vi "stepNhold.vi"() -> ()   [LabVIEW 2025]
panel:
  in  "T control mode":u16(ring)=4 items=["Tprobe", "Tsorb", "Fast Tsweep", "Skip T stable", "open loop", "Janis CCR", "PPMS"]
  in  "Motor control":enum16{"BLM motor", "IMS motor"}(ring)
  in  "stop dataacq":bool
  in  "T0 336":refnum<visa-resource-name>="GPIB0::12::INSTR"
  out "waiting (s)":dbl
  in  "meas time (s)":dbl=10.0
  in  "rate(T/min)":dbl=0.3 min=0.0
  in  "Power supply":T1(ring)
  in  "Exp. Mode":u16(ring)=1 items=["T sweep", "H sweep", "Angle sweep", "Other"]
  in  "Pass":bool
  in  "NML Data Acquisition VI":string(combo)="NML Data Acquisition-New.vi"
  out "stable":bool
  out "Reading":dbl=-999.99 format="%#_4g"
  out "done":i32
  in  "Finish":bool
  out "On Target":bool=TRUE
  in  "Target error":dbl=0.002 format="%#_13g"
  in  "timeout (s)":dbl=600.0
  out "time passed (s)":dbl format="%#_4g"
  out "status":string="Temp reached. Wait for stability"
  out "completed":bool
  out "table":dbl[][](array[numeric])=[[0.01, 0.41], [0.05, 0.32], [0.1, 0.33], [6.0, 2.0], [8.0, 2.0], [10.0, 2.0], [14.0, 2.0], [15.0, 2.0], [16.0, 2.0], [17.0, 2.0], [18.0, 2.0], [19.0, 2.0], [20.0, 2.0], [21.0, 2.0], [25.0, 1.0], [26.0, 2.0], [28.0, 2.0], [30.0, 2.0], [28.0, 2.0], [26.0, 2.0], [25.0, 2.0], [21.0, 1.0], [20.0, 2.0], [19.0, 2.0], [18.0, 2.0], [17.0, 2.0], [16.0, 2.0], [15.0, 2.0], [14.0, 2.0], [11.0, 1.0], [10.0, 2.0], [8.0, 2.0], [6.0, 2.0], [4.0, 2.0], [2.0, 2.0], [0.0, 2.0]]
  in  "Set T, wait (m)":string="0.01 0.41\n0.05 0.32\n0.1 0.33\n6 2\n8 2\n10 2\n14 2\n15 2\n16 2\n17 2\n18 2\n19 2\n20 2\n21 2\n25 1\n26 2\n28 2\n30 2\n28 2\n26 2\n25 2\n21 1\n20 2\n19 2\n18 2\n17 2\n16 2\n15 2\n14 2\n11 1\n10 2\n8 2\n6 2\n4 2\n2 2\n0 2" caption="Set Field(T), rate(T/min) (defualt rate: first row value)"
  in  "Use\nTable":bool
  in  "stable wait":dbl=10.0
  out "Target value":dbl=-1000.0
  in  "step":dbl=0.05
  in  "Final Target":dbl=1.0
  in  "Initial Target":dbl
  # "Step and Hold temperature, field or angle.\nData will be collected only when 'hold' state.\n\nField and Angle: There is no stability check\nTemp: Tcheck.vi check the stability.\n\nTiming\nstable wait: waiting time after 'hold' condition is met.\nmeas time (s): duration for data collection.\ntimeout (s): max time allowed to reach 'hold' condition."
  # "(s)"
  # "If ON, when the final target is reached,\ndata acq will be stopped\nand the data will be saved\n\nOtherwise, it will be paused."
  # "Txb: T's (0, hot, col) with heater off\nTxh: T's with heater on"
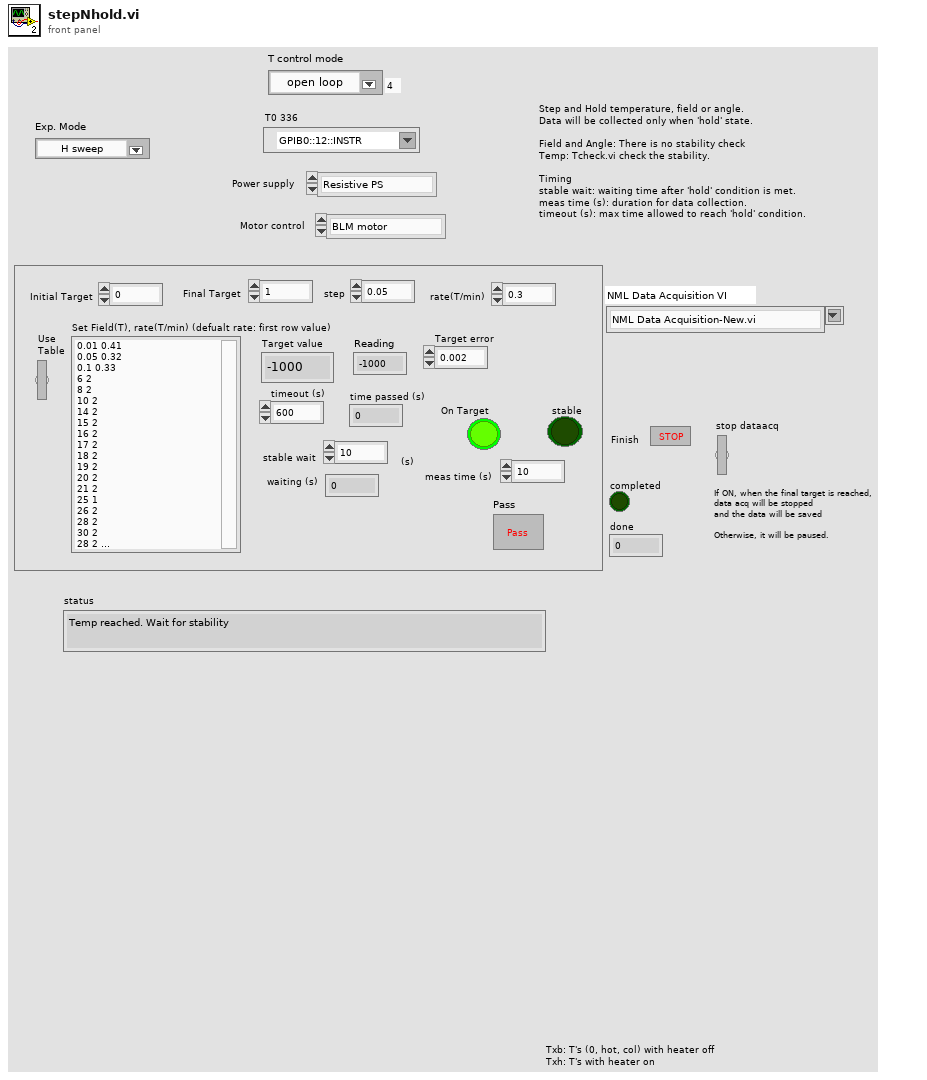
[diagram p1: front panel]
types:
  T1 = enum16{"Resistive PS", "SCM2 PS", "SCM1 PS", "Generic PS", "PPMS"}
  T2 = enum32{"New", "Stop", "Trigger", "Delta Trigger", "Run", "Pause"}
  T3 = enum32{"New", "Stop", "Trigger", "Delta Trigger", "Run", "Pause", "comments", "Started?"}
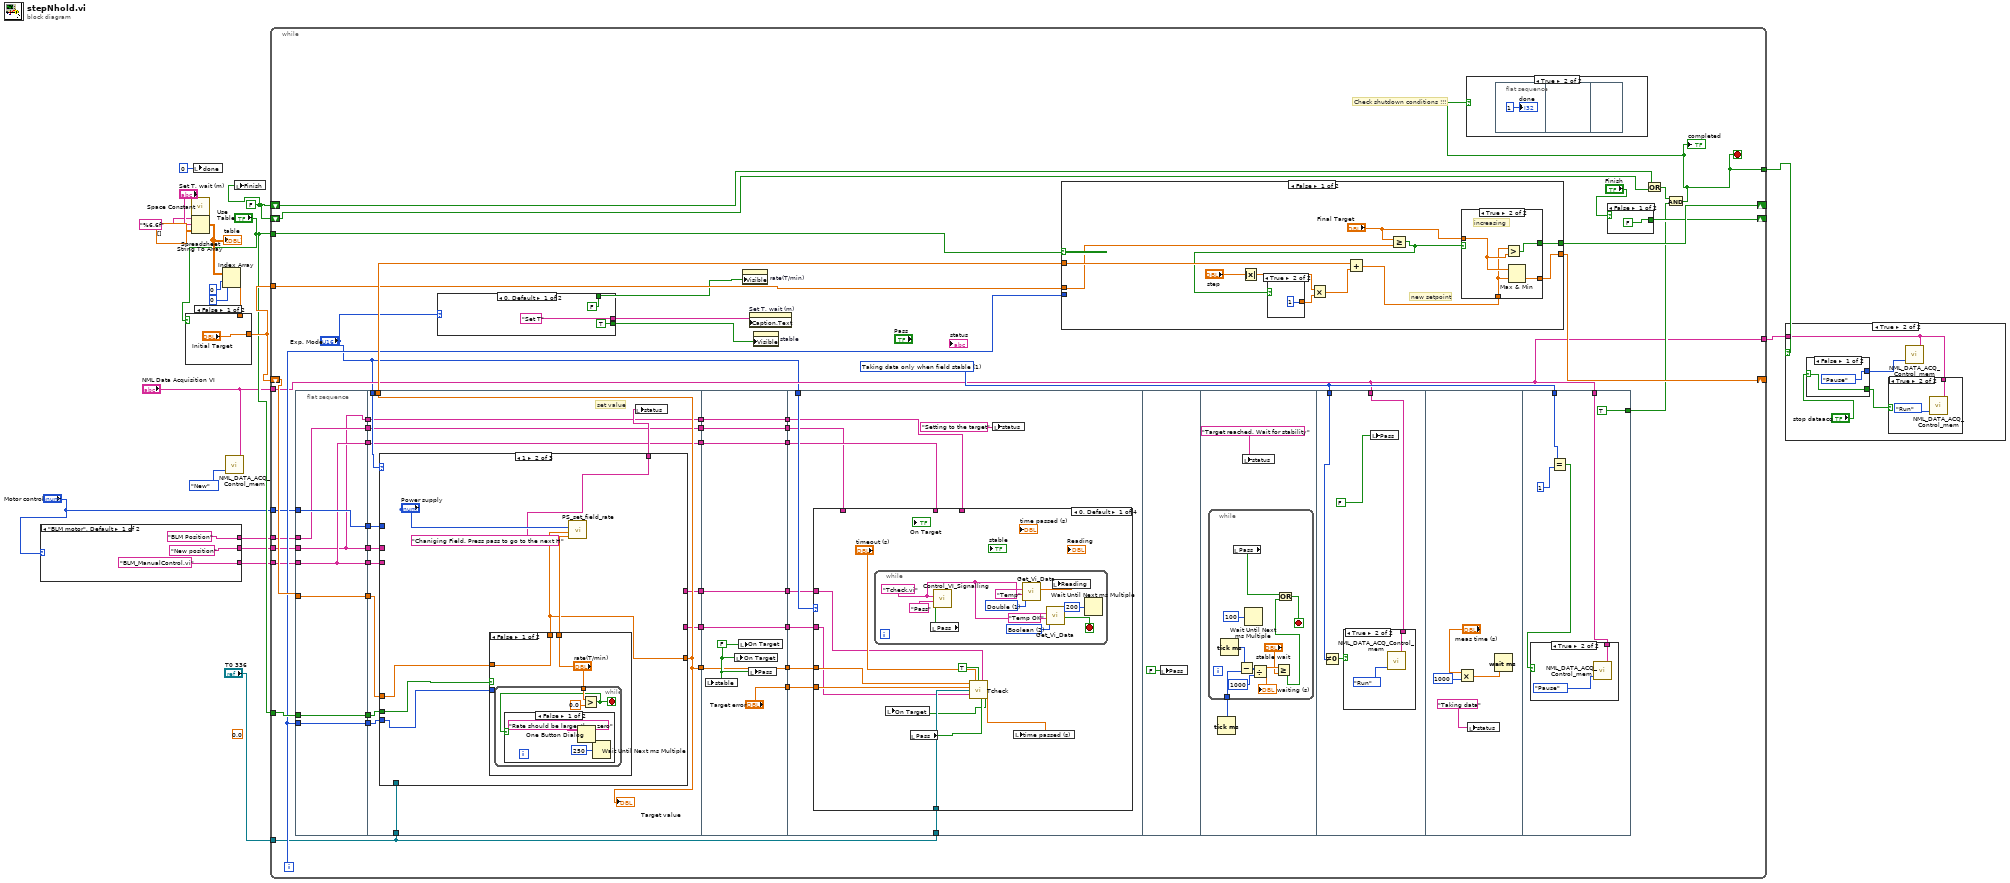
[diagram p0: block diagram]
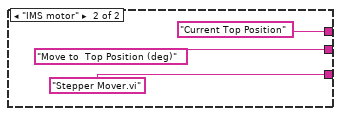
[diagram p2: hidden frame]
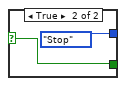
[diagram p5: hidden frame]
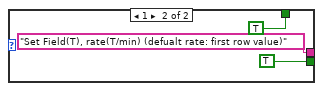
[diagram p7: hidden frame]
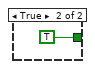
[diagram p9: hidden frame]
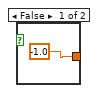
[diagram p10: hidden frame]
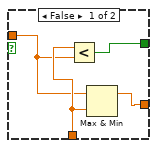
[diagram p11: hidden frame]
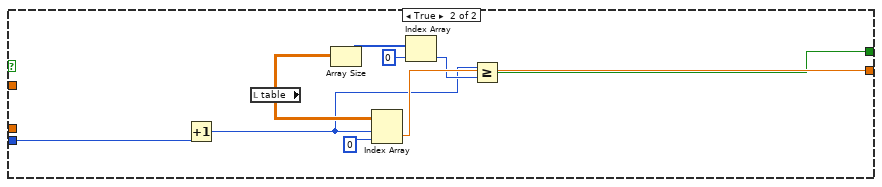
[diagram p12: hidden frame]
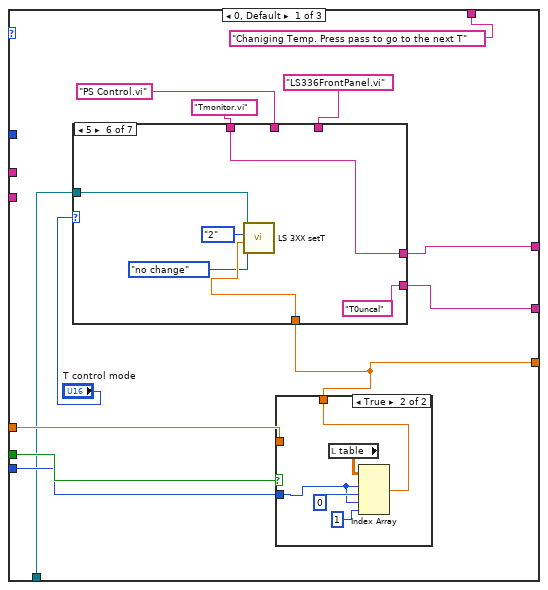
[diagram p13: hidden frame]
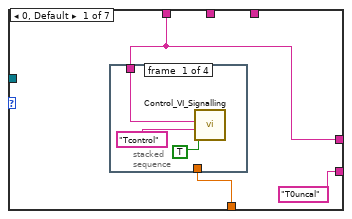
[diagram p14: hidden frame]
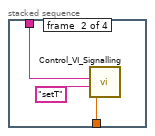
[diagram p15: hidden frame]
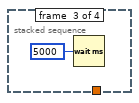
[diagram p16: hidden frame]
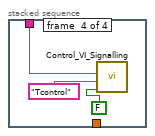
[diagram p17: hidden frame]
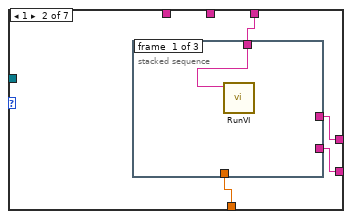
[diagram p18: hidden frame]
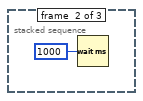
[diagram p19: hidden frame]
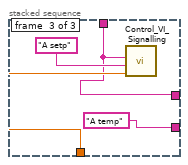
[diagram p20: hidden frame]
diagram:
  (unwired) 0.0 ("setT")
  w11 = FALSE
  n1 = case shown="\"BLM motor\", Default" "Motor control" {
    tunnel: ["BLM_ManualControl.vi" ("Target VI name") "Stepper Mover.vi" ("Target VI name")] -> w5
    tunnel: ["New position" ("Control Name") "Move to  Top Position (deg)" ("Control Name")] -> w4
    tunnel: ["BLM Position" "Current Top Position"] -> w2
    frame "BLM motor", Default {
    }
    frame "IMS motor" {
    }
  }
  n2 = call <vilib>:"Space Constant.vi"() -> ("String"=w17:string)
  n3 = Spreadsheet String To Array(delimiter (Tab)=w17, format string="%6.6f", spreadsheet string="Set T, wait (m)", array type (2D Dbl)=dbl[][] []) -> (array=w16:dbl[][])
  "table" <- w16
  n4 = local write "done"(0 ("done")) -> ()
  n5 = Index Array(array=w16, index (row)=0, index (col)=0 ("disabled index (col)")) -> (element=w13:dbl)
  n6 = case shown="False" "Use\nTable" {
    tunnel: ["Initial Target" w29] -> w21
    tunnel: w13 -> [_ w29]
    frame False {
    }
    frame True {
    }
  }
  n7 = call "NML_DATA_ACQ_Control_mem.vi"("Enum"=T2."New", "NML Data Acquisition VI"="NML Data Acquisition VI") -> ()  [unwired: 4 in, 1 out]
  n8 = local write "Finish"(w11) -> ()
  n9 = while {
    shift-right: [w75] -> _
    shift-left: w21 -> [w77]
    tunnel: w21 -> [w74]
    tunnel: "Use\nTable" -> [w73]
    tunnel: "Use\nTable" -> [w72]
    shift-right: [w70] -> _
    shift-left: w11 -> [w66]
    shift-right: [w67] -> _
    shift-left: w11 -> [w65]
    tunnel: "NML Data Acquisition VI" -> [w54]
    tunnel: [w55] -> w7
    tunnel: [w54] -> w6
    tunnel: w5 -> [w50]
    tunnel: w4 -> [w49]
    tunnel: "Motor control" -> [w46]
    tunnel: w2 -> [w42]
    tunnel: "T0 336" -> [w34]
    i -> [w71]
    stop <- w55 stop-if-true
    w69 = u16 1 items=["No interrupt", "Taking data only when field stable", "Taking data always"] ("Data acqusition ? (Run and Pause)")
    # "Check shutdown conditions !!!"
    n10 = flat-sequence {
      tunnel: w71 -> [w121]
      tunnel: w72 -> [w122]
      tunnel: w77 -> [w123]
      tunnel: [w123] -> w58
      tunnel: [w122] -> w57
      tunnel: [w121] -> w56
      tunnel: [w119] -> w51
      tunnel: w50 -> [w119]
      tunnel: w49 -> [w117]
      tunnel: [w117] -> w48
      tunnel: [w120] -> w47
      tunnel: w46 -> [w120]
      tunnel: [w119] -> w43
      tunnel: w42 -> [w118]
      tunnel: [w118] -> w41
      tunnel: [w117] -> w36
      tunnel: [w132] -> w76
      tunnel: "Exp. Mode" -> [w134]
      tunnel: w58 -> [w136]
      tunnel: w57 -> [w138]
      tunnel: w56 -> [w137]
      tunnel: w34 -> [w133]
      tunnel: [w132] -> w53
      tunnel: w51 -> [w131]
      tunnel: w48 -> [w130]
      tunnel: w47 -> [w129]
      tunnel: [w128] -> w44
      tunnel: w43 -> [w128]
      tunnel: w41 -> [w127]
      tunnel: [w127] -> w40
      tunnel: [w126] -> w37
      tunnel: w36 -> [w126]
      tunnel: [w125] -> w33
      tunnel: [w124] -> w31
      tunnel: ["Target error"] -> w64
      tunnel: w53 -> [w270]
      tunnel: [w270] -> w52
      tunnel: [w269] -> w45
      tunnel: w44 -> [w269]
      tunnel: w40 -> [w268]
      tunnel: [w268] -> w39
      tunnel: [w267] -> w38
      tunnel: w37 -> [w267]
      tunnel: w33 -> [w266]
      tunnel: [w266] -> w32
      tunnel: w31 -> [w265]
      tunnel: [w265] -> w30
      tunnel: "Exp. Mode" -> [w282]
      tunnel: w64 -> [w281]
      tunnel: w52 -> [w279]
      tunnel: w45 -> [w278]
      tunnel: w39 -> [w277]
      tunnel: w38 -> [w276]
      tunnel: w34 -> [w275]
      tunnel: w32 -> [w274]
      tunnel: w30 -> [w273]
      tunnel: w69 -> [w362]
      tunnel: w54 -> [w361]
      tunnel: w69 -> [w375]
      tunnel: [TRUE] -> w59
      tunnel: w54 -> [w371]
      frame #0 {
      }
      frame #1 {
        # "set value"
        n11 = case shown="1" w134 {
          tunnel: w138 -> [w150 w215 w246]
          tunnel: w137 -> [w149 w218 w247]
          tunnel: w136 -> [w148 w214 w245]
          tunnel: [w144 w213 w243] -> w132
          tunnel: ["Chaniging Temp. Press pass to go to the next T" ("status") "Chaniging Field. Press pass to go to the next H" ("status") "Chaniging angle. Press pass to go to the next angle" ("status")] -> w135
          tunnel: w133 -> [w143 _ _]
          tunnel: w131 -> [_ _ w241]
          tunnel: w130 -> [_ _ w240]
          tunnel: w129 -> [_ _ w239]
          tunnel: [w140 _ _] -> w125
          tunnel: [w139 _ _] -> w124
          frame 0, Default {
            n12 = case shown="True" w150 {
              tunnel: [w206 w210] -> w144
              tunnel: w149 -> [_ w208]
              tunnel: w148 -> [w206 _]
              frame False {
              }
              frame True {
                n13 = local read "table"() -> (w211:dbl[][])
                n14 = Index Array(array=w211, index (row) #1=w208, index (col) #1=0 ("disabled index (row)"), index (row) #2=w208, index (col) #2=1 ("disabled index (col)")) -> (element #1=w210:dbl)  [unwired: 1 out]
              }
            }
            n15 = case shown="5" "T control mode" {
              tunnel: w144 -> [w151 w167 _ _ w175 w193 w199]
              tunnel: ["T0uncal" ("VI name") w166 _ _ "T0uncal" ("VI name") "T0uncal" ("VI name") w198] -> w139
              tunnel: "Tmonitor.vi" ("VI name") -> [w152 _ _ _ w174 w194 _]
              tunnel: [w152 w165 _ _ w174 w194 w197] -> w140
              tunnel: "LS336FrontPanel.vi" ("Target VI name") -> [_ w164 _ _ _ _ _]
              tunnel: w143 -> [_ _ _ _ _ w191 _]
              tunnel: "PS Control.vi" ("VI name") -> [_ _ _ _ _ _ w196]
              frame 0, Default {
                n16 = stacked-sequence {
                  tunnel: w152 -> [w155 w158 _ w163]
                  tunnel: w151 -> [_ w157 _ _]
                  frame #0 {
                    n17 = call "Control_VI_Signalling.vi"("Input Value"=TRUE ("Pass"), "Control Name"="Tcontrol", "Target VI name"=w155) -> ()  [unwired: 8 in, 1 out]
                  }
                  frame #1 {
                    n18 = call "Control_VI_Signalling.vi"("Input Value"=w157, "Control Name"="setT", "Target VI name"=w158) -> ()  [unwired: 8 in, 1 out]
                  }
                  frame #2 {
                    n19 = Wait (ms)(milliseconds to wait=u32 5000) -> ()  [unwired: 1 out]
                  }
                  frame #3 {
                    n20 = call "Control_VI_Signalling.vi"("Input Value"=FALSE ("Pass"), "Control Name"="Tcontrol", "Target VI name"=w163) -> ()  [unwired: 8 in, 1 out]
                  }
                }
              }
              frame 1 {
                n21 = stacked-sequence {
                  tunnel: w167 -> [_ _ w172]
                  tunnel: [_ _ "A temp" ("VI name")] -> w166
                  tunnel: [_ _ w170] -> w165
                  tunnel: w164 -> [w168 _ w170]
                  frame #0 {
                    n22 = call "RunVI.vi"("String"=w168) -> ()  [unwired: 10 in, 1 out]
                  }
                  frame #1 {
                    n23 = Wait (ms)(milliseconds to wait=u32 1000) -> ()  [unwired: 1 out]
                  }
                  frame #2 {
                    n24 = call "Control_VI_Signalling.vi"("Input Value"=w172, "Control Name"="A setp", "Target VI name"=w170) -> ()  [unwired: 8 in, 1 out]
                  }
                }
              }
              frame 2 {
              }
              frame 3 {
              }
              frame 4 {
                n25 = stacked-sequence {
                  tunnel: w174 -> [w177 w181 w184 _ w188]
                  tunnel: w175 -> [w178 _ _ _ _]
                  frame #0 {
                    n26 = call "Control_VI_Signalling.vi"("Input Value"=w178, "Control Name"="mc current", "Target VI name"=w177) -> ()  [unwired: 8 in, 1 out]
                  }
                  frame #1 {
                    n27 = call "Control_VI_Signalling.vi"("Input Value"=1 ("disabled index (col)"), "Control Name"="control mode", "Target VI name"=w181) -> ()  [unwired: 8 in, 1 out]
                  }
                  frame #2 {
                    n28 = call "Control_VI_Signalling.vi"("Input Value"=TRUE ("Pass"), "Control Name"="Tcontrol", "Target VI name"=w184) -> ()  [unwired: 8 in, 1 out]
                  }
                  frame #3 {
                    n29 = Wait (ms)(milliseconds to wait=u32 4000) -> ()  [unwired: 1 out]
                  }
                  frame #4 {
                    n30 = call "Control_VI_Signalling.vi"("Input Value"=FALSE ("Pass"), "Control Name"="Tcontrol", "Target VI name"=w188) -> ()  [unwired: 8 in, 1 out]
                  }
                }
              }
              frame 5 {
                n31 = call "LS 3XX setT.vi"("power"=enum16{"no change", "off", "low", "med", "high"}."no change", "setT"=w193, "loop"=enum16{"1", "2"}."2", "GPIB"=w191) -> ()  [unwired: 8 in]
              }
              frame 6 {
                n32 = stacked-sequence {
                  tunnel: w199 -> [_ _ w204]
                  tunnel: [_ _ "Tppms" ("VI name")] -> w198
                  tunnel: [_ _ w202] -> w197
                  tunnel: w196 -> [w200 _ w202]
                  frame #0 {
                    n33 = call "RunVI.vi"("String"=w200) -> ()  [unwired: 10 in, 1 out]
                  }
                  frame #1 {
                    n34 = Wait (ms)(milliseconds to wait=u32 1000) -> ()  [unwired: 1 out]
                  }
                  frame #2 {
                    n35 = call "Control_VI_Signalling.vi"("Input Value"=w204, "Control Name"="set T", "Target VI name"=w202) -> ()  [unwired: 8 in, 1 out]
                  }
                }
              }
            }
          }
          frame 1 {
            n36 = case shown="False" w215 {
              tunnel: ["rate(T/min)" w227] -> w216
              tunnel: w218 -> [_ w232]
              tunnel: [w220 w230] -> w213
              tunnel: w214 -> [w220 _]
              frame False {
                n37 = while {
                  tunnel: "rate(T/min)" -> [w223]
                  stop <- w221 stop-if-true
                  n38 = Greater?(x=w223, y=0.0) -> (0:w221:bool)
                  n39 = case shown="False" w221 {
                    frame False {
                      n40 = One Button Dialog(message="Rate should be larger than zero") -> ()  [unwired: 1 in, 1 out]
                      n41 = Wait Until Next ms Multiple(millisecond multiple=u32 250) -> ()  [unwired: 1 out]
                    }
                    frame True {
                    }
                  }
                }
              }
              frame True {
                n42 = local read "table"() -> (w226:dbl[][])
                n43 = Index Array(array=w226, index (row) #1=w232, index (col) #1=0 ("disabled index (row)"), index (row) #2=w232, index (col) #2=1 ("disabled index (col)")) -> (element #1=w230:dbl, element #2=w228:dbl)
                n44 = Not Equal To 0?(x=w228) -> (x != 0?=w229:bool)
                n45 = case shown="False" w229 {
                  tunnel: [w234 w238] -> w227
                  tunnel: w228 -> [_ w238]
                  tunnel: w226 -> [w237 _]
                  frame False {
                    n46 = Index Array(array=w237, index (row)=0, index (col)=1 ("disabled index (col)")) -> (element=w234:dbl)
                  }
                  frame True {
                  }
                }
              }
            }
            n47 = call "PS_set_field_rate.vi"("ramping rate"=w216, "set point"=w213, "Power supply"="Power supply") -> ()  [unwired: 1 in]
          }
          frame 2 {
            n48 = case shown="True" w246 {
              tunnel: w247 -> [_ w258]
              tunnel: [w252 w256] -> w243
              tunnel: w245 -> [w252 _]
              frame False {
              }
              frame True {
                n49 = local read "table"() -> (w253:dbl[][])
                n50 = Index Array(array=w253, index (row) #1=w258, index (col) #1=0 ("disabled index (row)"), index (row) #2=w258, index (col) #2=1 ("disabled index (col)")) -> (element #1=w256:dbl, element #2=w254:dbl)
                n51 = Not Equal To 0?(x=w254) -> (x != 0?=w255:bool)
                n52 = case shown="False" w255 {
                  tunnel: [w260 w264] -> _
                  tunnel: w254 -> [_ w264]
                  tunnel: w253 -> [w263 _]
                  frame False {
                    n53 = Index Array(array=w263, index (row)=0, index (col)=1 ("disabled index (col)")) -> (element=w260:dbl)
                  }
                  frame True {
                  }
                }
              }
            }
            n54 = call "Control_VI_Signalling.vi"("Input Value"=w243, "Control Name"=w240, "Target VI name"=w241) -> ("error out"=w242:errorcluster)  [unwired: 8 in]
            n55 = case shown="\"BLM motor\", Default" w239 {
              tunnel: w242 -> [w249 _]
              tunnel: w241 -> [w248 _]
              frame "BLM motor", Default {
                n56 = call "Control_VI_Signalling.vi"("error in (no error)"=w249, "Input Value"=TRUE ("Use\nTable"), "Control Name"="Run", "Target VI name"=w248) -> ()  [unwired: 7 in, 1 out]
              }
              frame "IMS motor" {
              }
            }
          }
        }
        "Target value" <- w132
        n57 = local write "status"(w135) -> ()
      }
      frame #2 {
        w271 = FALSE ("Pass")
        n58 = local write "stable"(w271) -> ()
        n59 = local write "On Target"(w271) -> ()
        n60 = local write "On Target"(w271) -> ()
        n61 = local write "Pass"(w271) -> ()
      }
      frame #3 {
        n62 = case shown="0, Default" w282 {
          tunnel: w279 -> [w292 _ _ _]
          tunnel: w281 -> [w291 w304 w328 _]
          tunnel: w275 -> [w290 _ _ _]
          tunnel: w278 -> [_ _ w326 _]
          tunnel: w277 -> [_ _ w325 _]
          tunnel: w276 -> [_ _ w324 _]
          tunnel: w274 -> [w284 _ _ _]
          tunnel: w273 -> [w283 _ _ _]
          frame 0, Default {
            n63 = while {
              stop <- w293 stop-if-true
              w300 = u16 2 items=["String", "Double", "Boolean", "Variant"] ("Data Type")
              w301 = u16 1 items=["String", "Double", "Boolean", "Variant"] ("Data Type")
              w297 = "Tcheck.vi" ("Target VI name")
              n64 = local read "Pass"() -> (w302:bool)
              n65 = call "Control_VI_Signalling.vi"("Input Value"=w302, "Control Name"="Pass", "Target VI name"=w297) -> ()  [unwired: 8 in, 1 out]
              n66 = call "Get_Vi_Data.vi"("Data Type"=w301, "VI name"=w297, "Control Name"="Temp" ("VI name")) -> ("Data (Double)"=w294:dbl)  [unwired: 4 in, 4 out]
              n67 = call "Get_Vi_Data.vi"("Data Type"=w300, "VI name"=w297, "Control Name"="Temp OK" ("VI name")) -> ("Boolean"=w293:bool)  [unwired: 4 in, 4 out]
              n68 = local write "Reading"(w294) -> ()
              n69 = Wait Until Next ms Multiple(millisecond multiple=u32 200) -> ()  [unwired: 1 out]
            }
            n70 = local read "Pass"() -> (w288:bool)
            n71 = call "Tcheck.vi"("TargetT"=w292, "timeout (s)"="timeout (s)", "Direct reading"=TRUE, "VI name"=w284, "target T\nDT error"=w291, "VISA resource name"=w290, "T to watch"=w283, "Pass"=w288) -> ("Temp close to\nTarget T"=w286:bool, "Temp"=w287:dbl)  [unwired: 4 in, 2 out]
            n72 = local write "On Target"(w286) -> ()
            n73 = local write "time passed (s)"(w287) -> ()
          }
          frame 1 {
            n74 = Tick Count (ms)() -> (millisecond timer value=w303:u32)
            n75 = while {
              tunnel: w304 -> [w312]
              tunnel: w303 -> [w309]
              tunnel: [w305] -> _
              stop <- w305 stop-if-true
              w317 = u16 1 items=["String", "Double", "Boolean", "Variant"] ("Data Type")
              w320 = "PS Control.vi" ("VI name")
              n76 = Wait Until Next ms Multiple(millisecond multiple=u32 200 ("200")) -> ()  [unwired: 1 out]
              n77 = Tick Count (ms)() -> (millisecond timer value=w310:u32)
              n78 = call "Get_Vi_Data.vi"("Data Type"=w317, "VI name"=w320, "Control Name"="Field [T]") -> ("error out"=w319:errorcluster, "Data (Double)"=w311:dbl)  [unwired: 4 in, 3 out]
              n79 = Subtract(x=w310, y=w309) -> (x-y=w308:u32)
              n80 = local write "Reading"(w311) -> ()
              n81 = call "Get_Vi_Data.vi"("error in (no error) 2"=w319, "Data Type"=w317, "VI name"=w320, "Control Name"="Setpoint [T]") -> ("Data (Double)"=w316:dbl)  [unwired: 3 in, 4 out]
              n82 = Divide(x=w308, y=u32 1000) -> (x/y=w306:dbl)
              n83 = Subtract(x=w316, y=w311) -> (x-y=w314:dbl)
              n84 = Absolute Value(x=w314) -> (abs(x)=w315:dbl)
              n85 = local write "time passed (s)"(w306) -> ()
              n86 = local read "Pass"() -> (w323:bool)
              n87 = Less?(x=w315, y=w312) -> (x < y?=w313:bool)
              n88 = Or(x=w313, y=w323) -> (x .or. y?=w305:bool)
              n89 = local write "On Target"(w305) -> ()
            }
          }
          frame 2 {
            n90 = Tick Count (ms)() -> (millisecond timer value=w327:u32)
            n91 = while {
              tunnel: w328 -> [_]
              tunnel: w327 -> [w336]
              tunnel: w326 -> [w331]
              tunnel: w325 -> [w330]
              tunnel: w324 -> [w329]
              stop <- w339 stop-if-true
              w344 = u16 1 items=["String", "Double", "Boolean", "Variant"] ("Data Type")
              n92 = Wait Until Next ms Multiple(millisecond multiple=u32 200 ("200")) -> ()  [unwired: 1 out]
              n93 = Tick Count (ms)() -> (millisecond timer value=w337:u32)
              n94 = call "Get_Vi_Data.vi"("Data Type"=w344, "VI name"=w331, "Control Name"=w330) -> ("error out"=w345:errorcluster, "Data (Double)"=w338:dbl)  [unwired: 4 in, 3 out]
              n95 = Subtract(x=w337, y=w336) -> (x-y=w335:u32)
              n96 = local write "Reading"(w338) -> ()
              n97 = call "Get_Vi_Data.vi"("error in (no error) 2"=w345, "Data Type"=w344, "VI name"=w331, "Control Name"=w329) -> ("Data (Double)"=w343:dbl)  [unwired: 3 in, 4 out]
              n98 = Divide(x=w335, y=u32 1000) -> (x/y=w333:dbl)
              n99 = Subtract(x=w343, y=w338) -> (x-y=w341:dbl)
              n100 = Absolute Value(x=w341) -> (abs(x)=w342:dbl)
              n101 = local write "time passed (s)"(w333) -> ()
              n102 = local read "Pass"() -> (w347:bool)
              n103 = Less?(x=w342, y=2.0) -> (x < y?=w340:bool)
              n104 = Or(x=w340, y=w347) -> (x .or. y?=w339:bool)
              n105 = local write "On Target"(w339) -> ()
            }
          }
          frame 3 {
          }
        }
        n106 = local write "status"("Setting to the target" ("status")) -> ()
      }
      frame #4 {
        n107 = local write "Pass"(FALSE ("Pass")) -> ()
      }
      frame #5 {
        n108 = Tick Count (ms)() -> (millisecond timer value=w349:u32)
        n109 = while {
          tunnel: w349 -> [w357]
          stop <- w351 stop-if-true
          n110 = Tick Count (ms)() -> (millisecond timer value=w358:u32)
          n111 = local read "Pass"() -> (w352:bool)
          n112 = Subtract(x=w358, y=w357) -> (x-y=w360:u32)
          n113 = Wait Until Next ms Multiple(millisecond multiple=u32 100) -> ()  [unwired: 1 out]
          n114 = Divide(x=w360, y=u32 1000) -> (x/y=w356:dbl)
          "waiting (s)" <- w356
          n115 = Greater Or Equal?(x=w356, y="stable wait") -> (x >= y?=w353:bool)
          n116 = Or(x=w352, y=w353) -> (x .or. y?=w351:bool)
        }
        n117 = local write "status"("Target reached. Wait for stability" ("status")) -> ()
      }
      frame #6 {
        n118 = Not Equal To 0?(x=w362) -> (x != 0?=w363:bool)
        n119 = case shown="True" w363 {
          tunnel: w361 -> [_ w365]
          frame False {
          }
          frame True {
            n120 = call "NML_DATA_ACQ_Control_mem.vi"("Enum"=T2."Run", "NML Data Acquisition VI"=w365) -> ()  [unwired: 4 in, 1 out]
          }
        }
        n121 = local write "Pass"(FALSE ("Pass")) -> ()
      }
      frame #7 {
        n122 = Multiply(x="meas time (s)", y=u32 1000) -> (x*y=w369:dbl)
        n123 = local write "status"("Taking data" ("status")) -> ()
        n124 = Wait (ms)(milliseconds to wait=w369) -> ()  [unwired: 1 out]
      }
      frame #8 {
        n125 = Equal?(x=w375, y=u16 1) -> (x = y?=w373:bool)
        n126 = case shown="True" w373 {
          tunnel: w371 -> [_ w376]
          frame False {
          }
          frame True {
            n127 = call "NML_DATA_ACQ_Control_mem.vi"("Enum"=T3."Pause", "NML Data Acquisition VI"=w376) -> ()  [unwired: 4 in, 1 out]
          }
        }
      }
    }
    n128 = case shown="0, Default" "Exp. Mode" {
      tunnel: ["Set T" ("Caption.Text") "Set Field(T), rate(T/min) (defualt rate: first row value)" ("Caption.Text")] -> w63
      tunnel: [TRUE ("Visible") TRUE ("Visible")] -> w62
      tunnel: [FALSE ("Visible") TRUE ("Visible")] -> w61
      frame 0, Default {
      }
      frame 1 {
      }
    }
    n129 = property on="rate(T/min)" class="DigNum (strict)"("Visible"=w61) -> ()  [unwired: 2 in, 2 out]
    n130 = property on="Set T, wait (m)" class="Str"("Caption.Text"=w63) -> ()  [unwired: 2 in, 2 out]
    n131 = property on="stable" class="Bool (strict)"("Visible"=w62) -> ()  [unwired: 2 in, 2 out]
    n132 = case shown="False" w73 {
      tunnel: w76 -> [w97 _]
      tunnel: [w96 w111] -> w70
      tunnel: [w94 w116] -> w75
      tunnel: w74 -> [w92 _]
      tunnel: w71 -> [_ w109]
      frame False {
        # "new setpoint"
        n133 = Absolute Value(x="step") -> (abs(x)=w90:dbl)
        n134 = Greater Or Equal?(x="Final Target", y=w92) -> (x >= y?=w88:bool)
        n135 = case shown="True" w88 {
          tunnel: [-1.0 ("x*y") u32 1 ("y")] -> w87
          frame False {
          }
          frame True {
          }
        }
        n136 = Multiply(x=w90, y=w87) -> (x*y=w89:dbl)
        n137 = Add(x=w97, y=w89) -> (x+y=w95:dbl)
        n138 = case shown="True" w88 {
          tunnel: w95 -> [w102 w105]
          tunnel: "Final Target" -> [w101 w106]
          tunnel: [w103 w107] -> w96
          tunnel: [w100 w104] -> w94
          frame False {
            n139 = Less?(x=w102, y=w101) -> (x < y?=w103:bool)
            n140 = Max & Min(x=w101, y=w102) -> (max(x,y)=w100:dbl)  [unwired: 1 out]
          }
          frame True {
            # "increasing"
            n141 = Greater?(x=w105, y=w106) -> (0:w107:bool)
            n142 = Max & Min(x=w106, y=w105) -> (min(x,y)=w104:dbl)  [unwired: 1 out]
          }
        }
      }
      frame True {
        n143 = Increment(x=w109) -> (x+1=w108:i32)
        n144 = local read "table"() -> (w115:dbl[][])
        n145 = Array Size(array=w115) -> (size(s)=w114:i32[])
        n146 = Index Array(array=w115, index (row)=w108, index (col)=0 ("disabled index (col)")) -> (element=w116:dbl)
        n147 = Index Array(array=w114, index=0) -> (element=w112:i32)
        n148 = Greater Or Equal?(x=w108, y=w112) -> (x >= y?=w111:bool)
      }
    }
    n149 = case shown="False" "Finish" {
      tunnel: [FALSE TRUE] -> w67
      frame False {
      }
      frame True {
      }
    }
    n150 = Or(x=w66, y=w65) -> (x .or. y?=w60:bool)
    n151 = And(x=w60, y=w59) -> (x .and. y?=w55:bool)
    "completed" <- w55
    n152 = case shown="True" w55 {
      frame False {
      }
      frame True {
        n153 = flat-sequence {
          frame #0 {
            "done" <- 1 ("done")
          }
          frame #1 {
          }
          frame #2 {
          }
        }
      }
    }
  }
  n154 = case shown="True" w7 {
    tunnel: w6 -> [_ w378]
    frame False {
    }
    frame True {
      n155 = case shown="False" "stop dataacq" {
        selector: "stop dataacq" -> [w384 w386]
        tunnel: [T3."Pause" ("Enum") T3."Stop" ("Enum")] -> w381
        tunnel: [w384 w386] -> w379
        frame False {
        }
        frame True {
        }
      }
      n156 = case shown="True" w379 {
        tunnel: w378 -> [_ w383]
        frame False {
        }
        frame True {
          n157 = call "NML_DATA_ACQ_Control_mem.vi"("Enum"=T3."Run", "NML Data Acquisition VI"=w383) -> ()  [unwired: 4 in, 1 out]
        }
      }
      n158 = call "NML_DATA_ACQ_Control_mem.vi"("Enum"=w381, "NML Data Acquisition VI"=w378) -> ()  [unwired: 4 in, 1 out]
    }
  }
